vi "Test Get Elements and Subelements.vi"(8 "Error In":errorcluster) -> ()   [LabVIEW 2018]
uses:
  <vilib>/Utility/traverseref.llb/TRef TravTarget.ctl
  <vilib>/Utility/traverseref.llb/VI Scripting - Traverse.lvlib
panel:
  out "objects count":i32
  out "while loops count":i32
  out "wires names in while loop":string[](array[string])
  out "loop tunnels elemnts count":i32
  out "LoopTunnel inside while loop":string[](array[string])
  out "Wires and connected ClassNames in for loop.":string[][](array[string])
  out "Objects[] in WhileLoop":string[](array[string])
  out "All Objects[]":string[](array[string])
  in  "vi path":path=path "C:/Users/lubo/Documents/LabView/LabVIEW-Universal-Transcriptor/Test/Examples For Parsing/Example Test 1.vi"
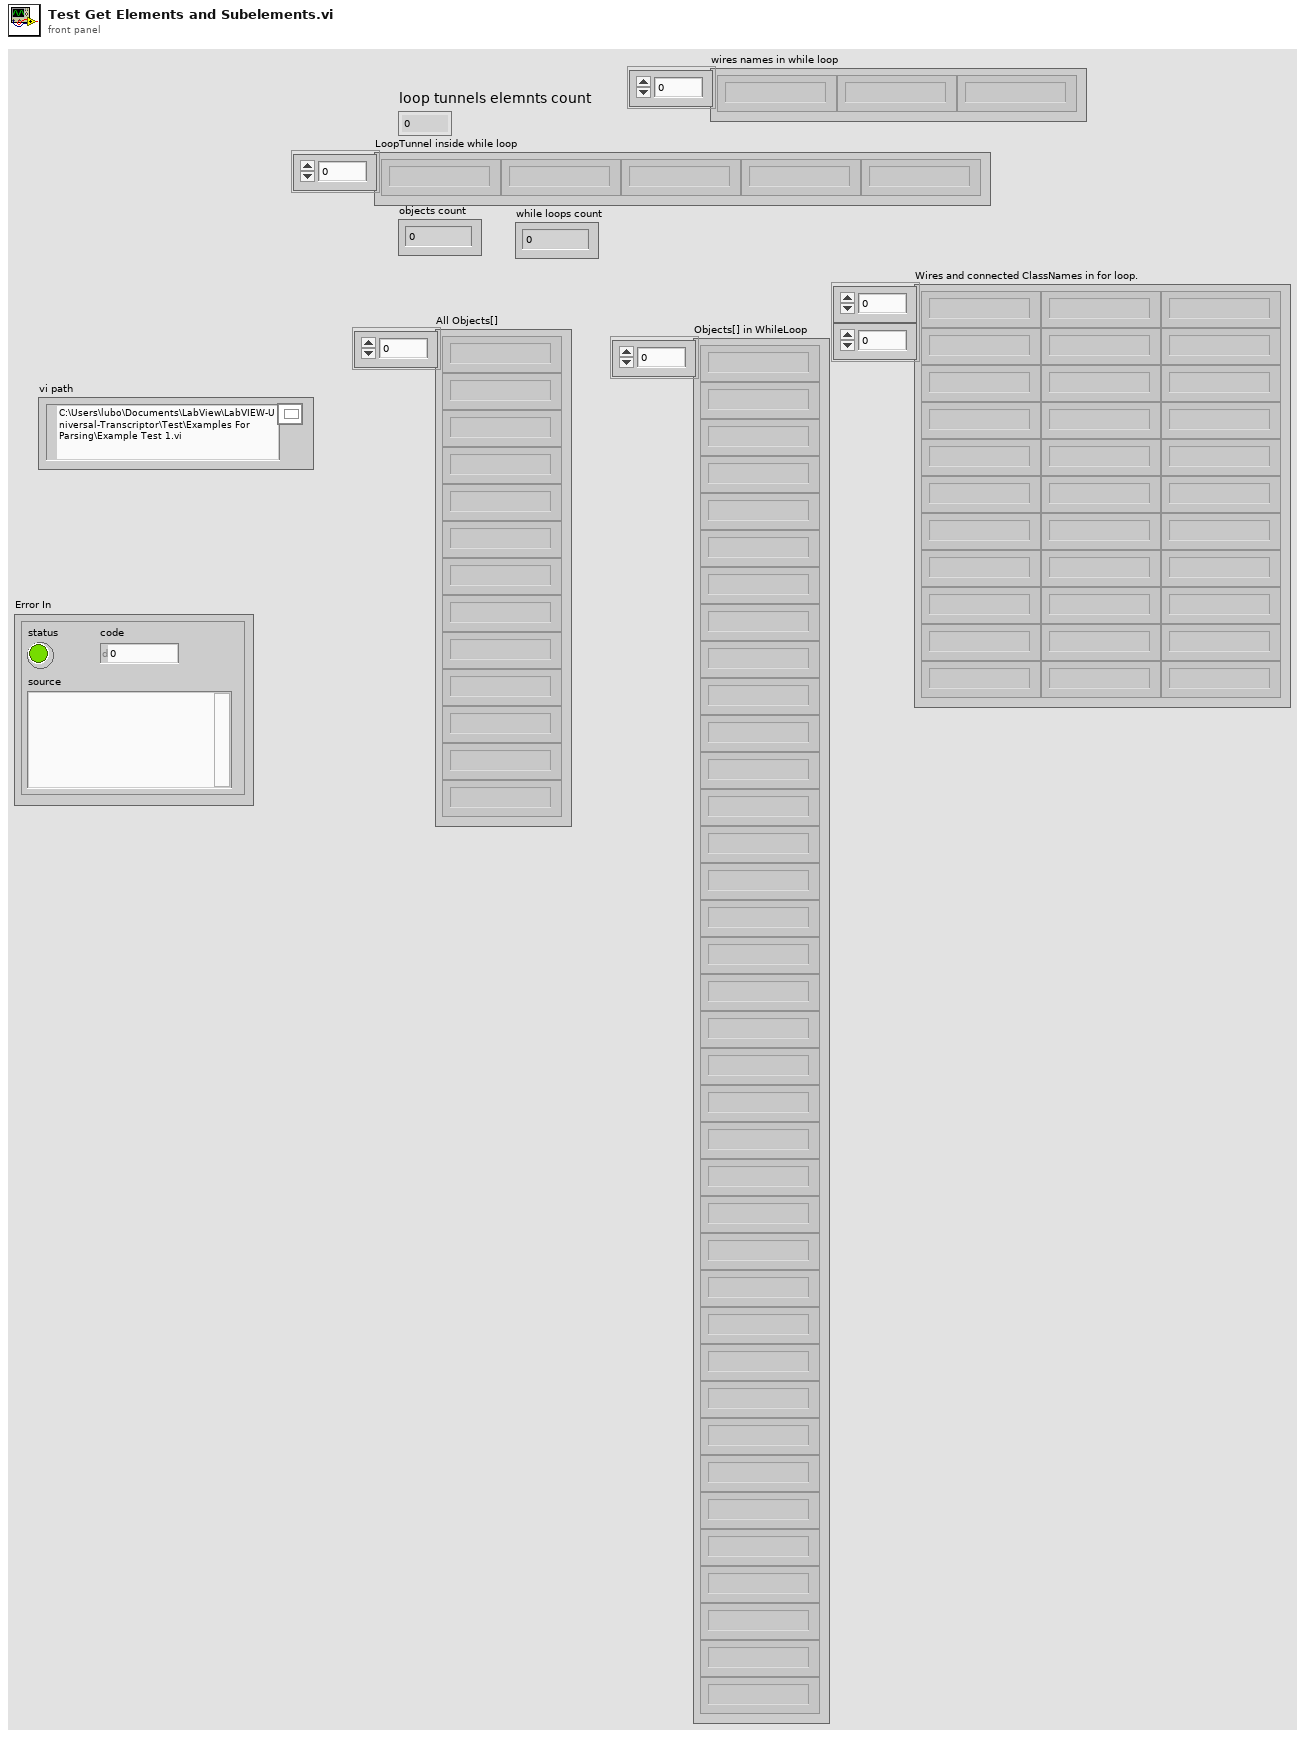
[diagram p1: front panel]
types:
  T1 = typedef "TRef TravTarget.ctl" = enum16{"FP", "BD", "Other"}
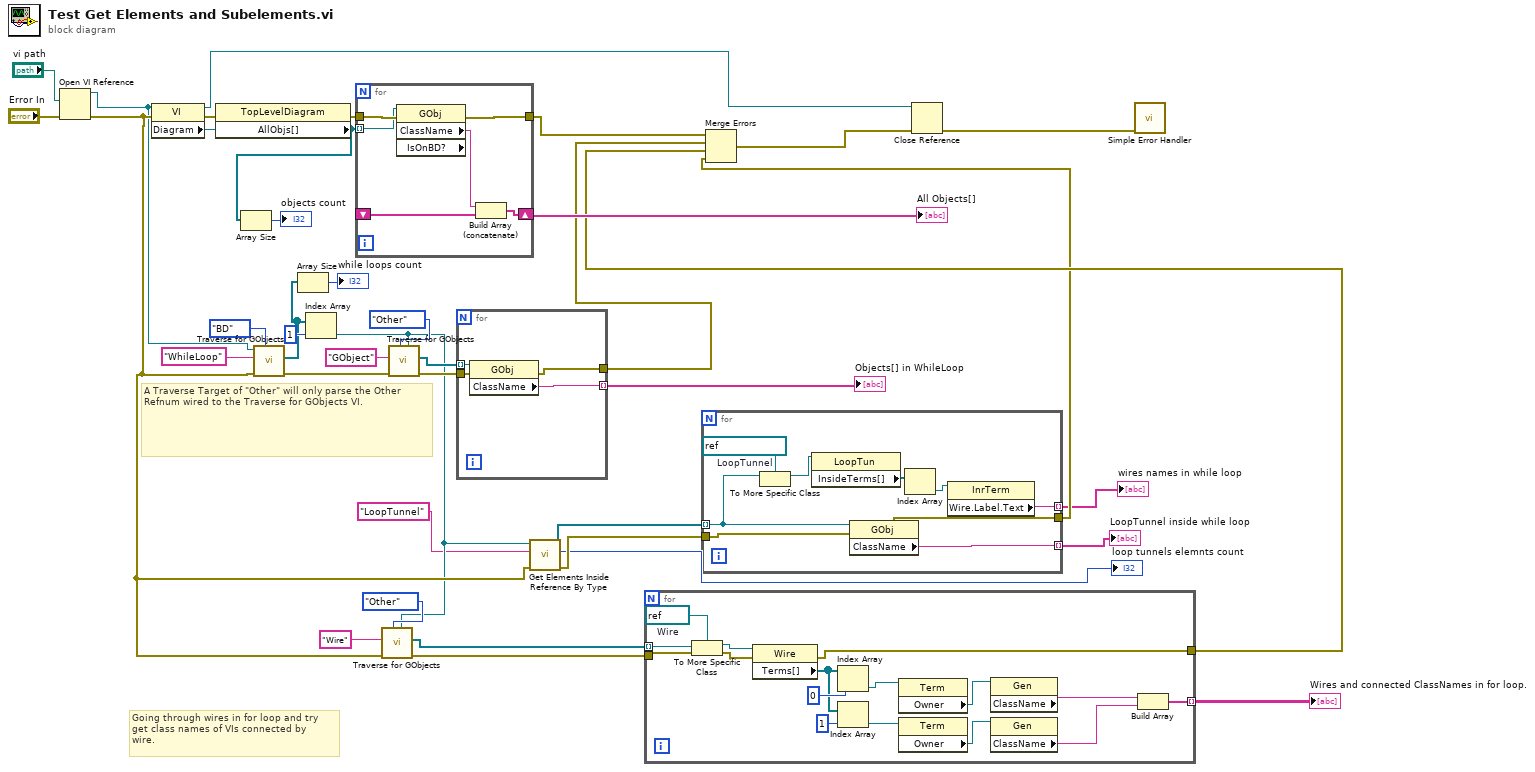
[diagram p0: block diagram]
diagram:
  # "Going through wires in for loop and try\nget class names of VIs connected by\nwire."
  # "A Traverse Target of \"Other\" will only parse the Other Refnum wired to the Traverse for GObjects VI."
  n1 = Open VI Reference(vi path="vi path", error in (no error)="Error In") -> (vi reference=w1:refnum<vi>, error out=w13:errorcluster)  [unwired: 4 in]
  n2 = property class="VI"(reference=w1, error in=w13) -> (reference out=w38:refnum<vi>, error out=w36:errorcluster, "Diagram"=w37:refnum<vi>)
  n3 = property class="TopLevelDiagram"(reference=w37, error in=w36) -> (error out=w34:errorcluster, "AllObjs[]"=w2:refnum<vi>[])  [unwired: 1 out]
  n4 = Array Size(array=w2) -> (size(s)=→"objects count":i32)
  n5 = call <vilib>:"Traverse for GObjects.vi"("Traverse Target"=TRef_TravTarget."BD", "error in (no error)"=w13, "Class Name"="WhileLoop", "VI Refnum"=w1) -> ("error out"=w31:errorcluster, "References"=w5:refnum<vi>[])  [unwired: 4 in, 2 out]
  n6 = Array Size(array=w5) -> (size(s)=→"while loops count":i32)
  n7 = Index Array(array=w5, index=1) -> (element=w10:refnum<vi>)
  n8 = for {
    tunnel: w34 -> [w46]
    tunnel: w2 -> [w45] mode=indexing
    shift-right: [w42] -> w33
    shift-left: _ -> [w43]
    tunnel: [w41] -> w24
    n9 = property class="GObj" props=["ClassName", "IsOnBD?"](reference=w45, error in=w46) -> (error out=w41:errorcluster, "ClassName"=w44:string)  [unwired: 2 out]
    n10 = Build Array (concatenate)(w44, w43) -> (w42:string[])
  }
  "All Objects[]" <- w33
  n11 = call <vilib>:"Traverse for GObjects.vi"("Other Refnum"=w10, "Traverse Target"=TRef_TravTarget."Other", "error in (no error)"=w13, "Class Name"="Wire") -> ("error out"=w20:errorcluster, "References"=w21:refnum<vi>[])  [unwired: 4 in, 2 out]
  n12 = call <vilib>:"Traverse for GObjects.vi"("Other Refnum"=w10, "Traverse Target"=TRef_TravTarget."Other", "error in (no error)"=w31, "Class Name"="GObject") -> ("error out"=w27:errorcluster, "References"=w26:refnum<vi>[])  [unwired: 4 in, 2 out]
  n13 = for {
    tunnel: w27 -> [w50]
    tunnel: w26 -> [w49] mode=indexing
    tunnel: [w48] -> w25 mode=indexing
    tunnel: [w47] -> w23
    n14 = property class="GObj"(reference=w49, error in=w50) -> (error out=w47:errorcluster, "ClassName"=w48:string)  [unwired: 1 out]
  }
  "Objects[] in WhileLoop" <- w25
  n15 = call "Get Elements Inside Reference By Type.vi"("error in (no error)"=w13, "filter element class name"="LoopTunnel", "element ref."=w10) -> ("error out"=w14:errorcluster, "elemnts count"=→"loop tunnels elemnts count":i32, "elements ref."=w11:refnum<vi>[])  [unwired: 6 in]
  n16 = for {
    tunnel: w20 -> [w64]
    tunnel: w21 -> [w65] mode=indexing
    tunnel: [w66] -> w17
    tunnel: [w56] -> w16 mode=indexing
    w63 = refnum<vi> refnum  # Wire
    n17 = To More Specific Class(target class=w63, reference=w65, error in=w64) -> (specific class reference=w62:refnum<vi>, error out=w61:errorcluster)
    n18 = property class="Wire"(reference=w62, error in=w61) -> (error out=w66:errorcluster, "Terms[]"=w51:refnum<vi>[])  [unwired: 1 out]
    n19 = Index Array(array=w51, index=0) -> (element=w58:refnum<vi>)
    n20 = Index Array(array=w51, index=1) -> (element=w57:refnum<vi>)
    n21 = property class="Term"(reference=w58) -> ("Owner"=w55:refnum<vi>)  [unwired: 1 in, 2 out]
    n22 = property class="Term"(reference=w57) -> ("Owner"=w54:refnum<vi>)  [unwired: 1 in, 2 out]
    n23 = property class="Gen"(reference=w55) -> ("ClassName"=w52:string)  [unwired: 1 in, 2 out]
    n24 = property class="Gen"(reference=w54) -> ("ClassName"=w53:string)  [unwired: 1 in, 2 out]
    n25 = Build Array(w52, w53) -> (w56:string[])
  }
  "Wires and connected ClassNames in for loop." <- w16
  n26 = for {
    tunnel: w14 -> [w75]
    tunnel: [w74] -> w12
    tunnel: w11 -> [w72] mode=indexing
    tunnel: [w73] -> w7 mode=indexing
    tunnel: [w67] -> w6 mode=indexing
    w71 = refnum<vi> refnum  # LoopTunnel
    n27 = To More Specific Class(target class=w71, reference=w72) -> (specific class reference=w70:refnum<vi>)  [unwired: 1 in, 1 out]
    n28 = property class="LoopTun"(reference=w70) -> ("InsideTerms[]"=w69:refnum<vi>[])  [unwired: 1 in, 2 out]
    n29 = property class="GObj"(reference=w72, error in=w75) -> (error out=w74:errorcluster, "ClassName"=w73:string)  [unwired: 1 out]
    n30 = Index Array(array=w69) -> (element=w68:refnum<vi>)  [unwired: 1 in]
    n31 = property class="InrTerm"(reference=w68) -> ("Wire.Label.Text"=w67:string)  [unwired: 1 in, 2 out]
  }
  "LoopTunnel inside while loop" <- w7
  "wires names in while loop" <- w6
  n32 = Merge Errors(w24, w23, w17, w12) -> (w22:errorcluster)
  n33 = Close Reference(reference=w38, error in (no error)=w22) -> (error out=w39:errorcluster)
  n34 = call <vilib>:"Simple Error Handler.vi"("error in (no error)"=w39) -> ()  [unwired: 4 in, 5 out]
